vi "Move Right To Joints.vi"(5 "Label":string, 6 "Wait (s)":dbl, 8 "error in":errorcluster, 9 "time":dbl=2.0, 10 "Goal":dbl[](array[numeric])) -> (0 "error out":errorcluster, 2 "Goal":dbl[](array[numeric]))   [LabVIEW 2013]
uses:
  ROS/Code/Console/Servers/ServerSubs/(nist) Arm Globals.vi
panel:
  # "All Joint motions\nare relative to BASE"
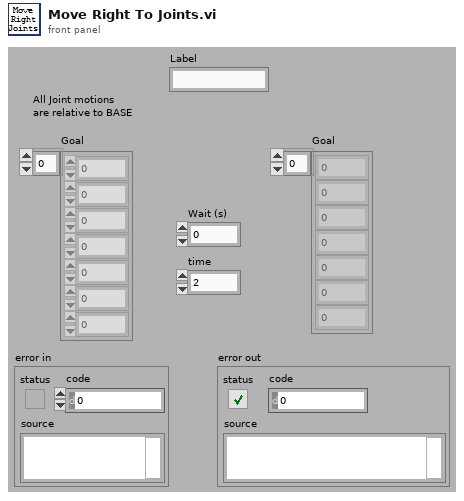
[diagram p1: front panel]
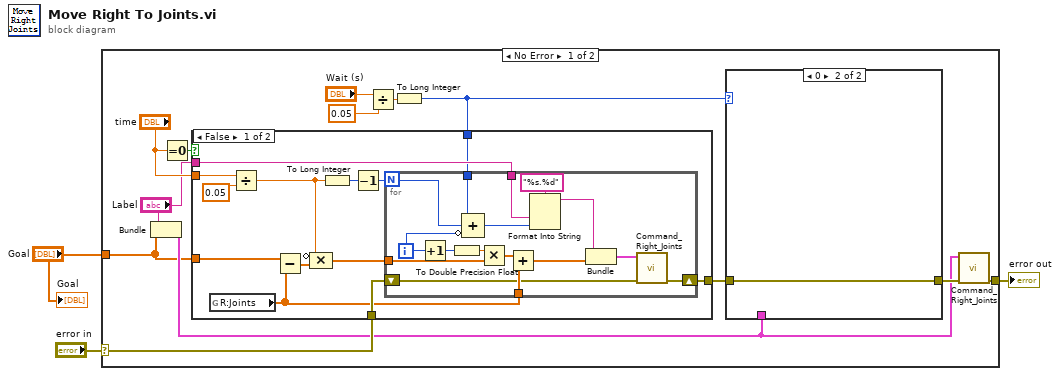
[diagram p0: block diagram]
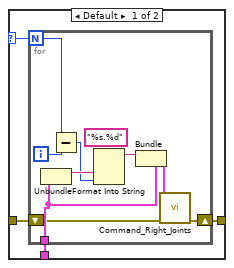
[diagram p2: hidden frame]
diagram:
  n1 = case shown="No Error" "error in" {
    selector: "error in" -> [w8 w61]
    tunnel: [w6 w61] -> w2
    tunnel: "Goal" -> [w4 _]
    frame No Error {
      n2 = Bundle("Label"="Label", "Goal"=w4) -> (w5:cluster{"Label":string, "Goal":dbl[]})  [unwired: 1 in]
      n3 = Equal To 0?(x="time") -> (x = 0?=w16:bool)
      n4 = Divide(x="Wait (s)", y=0.05) -> (x/y=w11:dbl)
      n5 = To Long Integer(number=w11) -> (32bit integer=w10:i32)
      n6 = case shown="False" w16 {
        tunnel: "Label" -> [w40 _]
        tunnel: w4 -> [w34 _]
        tunnel: "time" -> [w43 _]
        tunnel: w10 -> [w35 _]
        tunnel: [w32 w60] -> w9
        tunnel: w8 -> [w33 w60]
        frame False {
          n7 = global read "(nist) Arm Globals.vi" "R:Joints"() -> (w31:dbl[])
          n8 = Divide(x=w43, y=0.05) -> (x/y=w36:dbl)
          n9 = Subtract(x=w34, y=w31) -> (x-y=w37:dbl[])
          n10 = Compound Arithmetic op=MULTIPLY(invert w36, w37) -> (w38:dbl[])
          n11 = To Long Integer(number=w36) -> (32bit integer=w41:i32)
          n12 = Decrement(x=w41) -> (x-1=w39:i32)
          n13 = for {
            N: w39 -> [w59]
            tunnel: w38 -> [w56]
            tunnel: w40 -> [w54]
            tunnel: w35 -> [w51]
            tunnel: w31 -> [w49]
            shift-right: [w47] -> w32
            shift-left: w33 -> [w48]
            i -> [w58]
            n14 = Increment(x=w58) -> (x+1=w52:i32)
            n15 = To Double Precision Float(number=w52) -> (double precision float=w57:dbl)
            n16 = Compound Arithmetic op=ADD(w51, w59, invert w58) -> (w53:i32)
            n17 = Multiply(x=w57, y=w56) -> (x*y=w50:dbl[])
            n18 = Add(x=w50, y=w49) -> (x+y=w45:dbl[])
            n19 = Format Into String(format string="%s.%d", w54, w53) -> (resulting string=w46:string)  [unwired: 2 in, 1 out]
            n20 = Bundle(w46, w45) -> (w44:cluster{string, dbl[]})  [unwired: 1 in]
            n21 = call "Command_Right_Joints.vi"("error in"=w48, "Goal"=w44) -> ("error out"=w47:errorcluster)  [unwired: 6 in, 1 out]
          }
        }
        frame True {
        }
      }
      n22 = case shown="0" w10 {
        selector: w10 -> [w17 _]
        tunnel: w9 -> [w20 w30]
        tunnel: [w19 w30] -> w7
        tunnel: w5 -> [w18 _]
        frame Default {
          n23 = for {
            N: w17 -> [w29]
            tunnel: w18 -> [w24]
            shift-right: [w22] -> w19
            shift-left: w20 -> [w23]
            i -> [w28]
            (unwired) "%s.%d" ("format string")
            n24 = Unbundle(w24) -> ("Label"=w27:string)  [unwired: 1 out]
            n25 = Subtract(x=w29, y=w28) -> (x-y=w26:i32)
            n26 = Format Into String(w27, w26) -> (resulting string=w25:string)  [unwired: 3 in, 1 out]
            n27 = Bundle(cluster=w24, "Label"=w25) -> (w21:cluster{"Label":string, "Goal":dbl[]})  [unwired: 1 in]
            n28 = call "Command_Right_Joints.vi"("error in"=w23, "Goal"=w21) -> ("error out"=w22:errorcluster)  [unwired: 6 in, 1 out]
          }
        }
        frame 0 {
        }
      }
      n29 = call "Command_Right_Joints.vi"("error in"=w7, "Goal"=w5) -> ("error out"=w6:errorcluster)  [unwired: 6 in, 1 out]
    }
    frame Error {
    }
  }
  "error out" <- w2
  "Goal" <- "Goal"
